vi "GetParam.vi"(8 "error in (no error)":errorcluster caption="entrée d'erreur (pas d'erreur)", 11 "DictVectorizer.lvclass":refnum<class "DictVectorizer.lvclass">) -> (0 "error out":errorcluster caption="sortie d'erreur", 2 "DictVectorizer":T1={"dtype"="float", "separator"="=", "sparse"=TRUE, "sort"=TRUE}, 3 "DictVectorizer.lvclass":refnum<class "DictVectorizer.lvclass">)   [LabVIEW 2020, in "DictVectorizer.lvclass"]
doc: "Get Parameters"
uses:
  DictVectorizer.lvclass
  DictVectorizer.lvclass/DictVectorizer.ctl
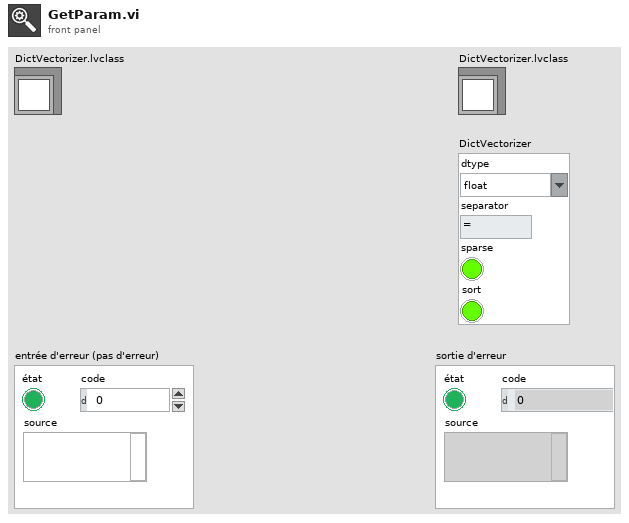
[diagram p1: front panel]
types:
  T1 = cluster{"dtype":string, "separator":string, "sparse":bool, "sort":bool}
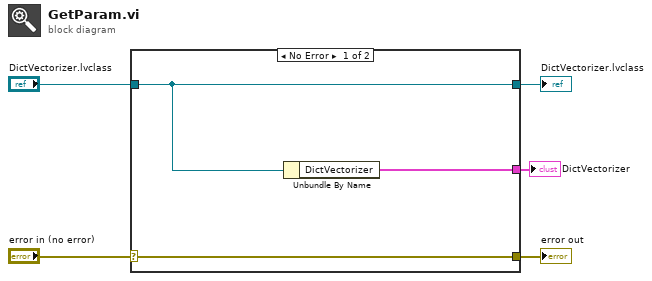
[diagram p0: block diagram]
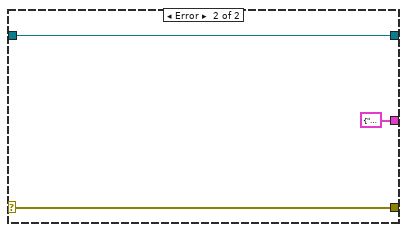
[diagram p2: hidden frame]
diagram:
  n1 = case shown="No Error" "error in (no error)" {
    selector: "error in (no error)" -> [w8 w10]
    tunnel: [w8 w10] -> w4
    tunnel: [w7 w11] -> w2
    tunnel: "DictVectorizer.lvclass" -> [w7 w11]
    tunnel: [w6 T1 {"dtype"="", "separator"="", "sparse"=FALSE, "sort"=FALSE} ("DictVectorizer")] -> w1
    frame No Error {
      n2 = Unbundle By Name(w7) -> ("DictVectorizer"=w6:T1)
    }
    frame Error {
    }
  }
  "error out" <- w4
  "DictVectorizer.lvclass" <- w2
  "DictVectorizer" <- w1
